vi "Close.vi"(8 "error in (no error)":errorcluster, 11 "Lambda Gen Plus in":refnum<class "Lambda Gen Plus.lvclass">) -> (0 "error out":errorcluster, 3 "Lambda Gen Plus out":refnum<class "Lambda Gen Plus.lvclass">)   [LabVIEW 2025, in "Power Supply.lvlib" / "Lambda Gen Plus.lvclass"]
uses:
  Lambda Gen Plus.lvclass
  Lambda Gen Plus.lvclass/Lambda Gen Plus.ctl
  58c1e3ef-388f-40d6-b018-f733c62815da.vi
  <instrlib>/TDK-Lambda G Series/TDK-Lambda G Series.lvlib
  PS Instrument/Power Supply Instrument.lvclass
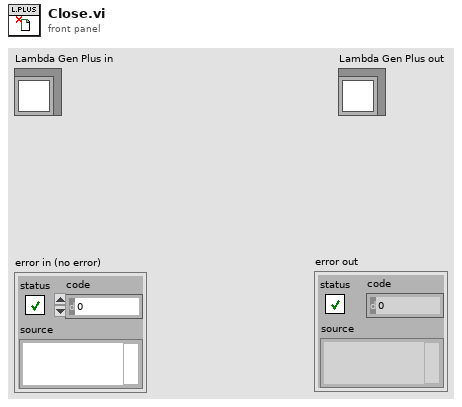
[diagram p1: front panel]
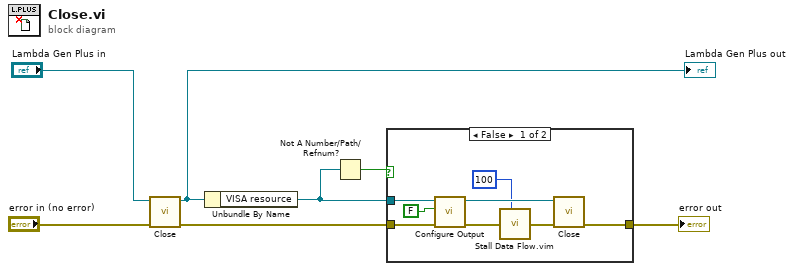
[diagram p0: block diagram]
diagram:
  n1 = call-parent <instrlib>:"Close.vi"("error in (no error)"="error in (no error)", "Power Supply Instrument in"="Lambda Gen Plus in") -> ("error out"=w3:errorcluster, "Power Supply Instrument out"=w1:refnum<class "Lambda Gen Plus.lvclass">)  [unwired: 8 in]
  "Lambda Gen Plus out" <- w1
  n2 = Unbundle By Name(w1) -> ("VISA resource"=w5:refnum<visa-resource-name>)
  n3 = Not A Number/Path/Refnum?(number/path/refnum=w5) -> (NaN/Path/Refnum?=w4:bool)
  n4 = case shown="False" w4 {
    tunnel: w3 -> [w14 w16]
    tunnel: [w15 w16] -> w6
    tunnel: w5 -> [w11 _]
    frame False {
      n5 = call <instrlib>:"Configure Output.vi"("error in (no error)"=w14, "Enable Output (False)"=FALSE, "VISA resource name"=w11) -> ("error out"=w13:errorcluster, "VISA resource name out"=w12:refnum<visa-resource-name>)  [unwired: 7 in]
      n6 = call "Stall Data Flow.vim"("value in"=w13, "milliseconds to wait"=u32 100) -> ("value out"=w9:errorcluster)  [unwired: 1 out]
      n7 = call <instrlib>:"Close.vi"("error in (no error)"=w9, "VISA resource name"=w12) -> ("error out"=w15:errorcluster)  [unwired: 9 in]
    }
    frame True {
    }
  }
  "error out" <- w6
